vi "MASS_FLOW_METER.vi"(0 "ESD":bool, 3 "Wire cut":bool) -> (1 "MFM Flow Rate (Discharge)":dbl, 2 "MFM Flow Rate (Inlet)":dbl, 4 "MFM Total Kg (Discharge)":dbl format="%#_9g", 5 "MFM Total Kg (Inlet)":dbl format="%#_9g")   [LabVIEW 2014]
panel:
  out "Inlet MFM Total Kg Trend (Kg)":dbl(graph)
  out "Discharge MFM Total Kg Trend (Kg)":dbl(graph)
  out "Inlet MFM Flow Rate Trend (Kg/m2)":dbl(graph)
  out "Discharge MFM Flow Rate Trend (Kg/m2)":dbl(graph)
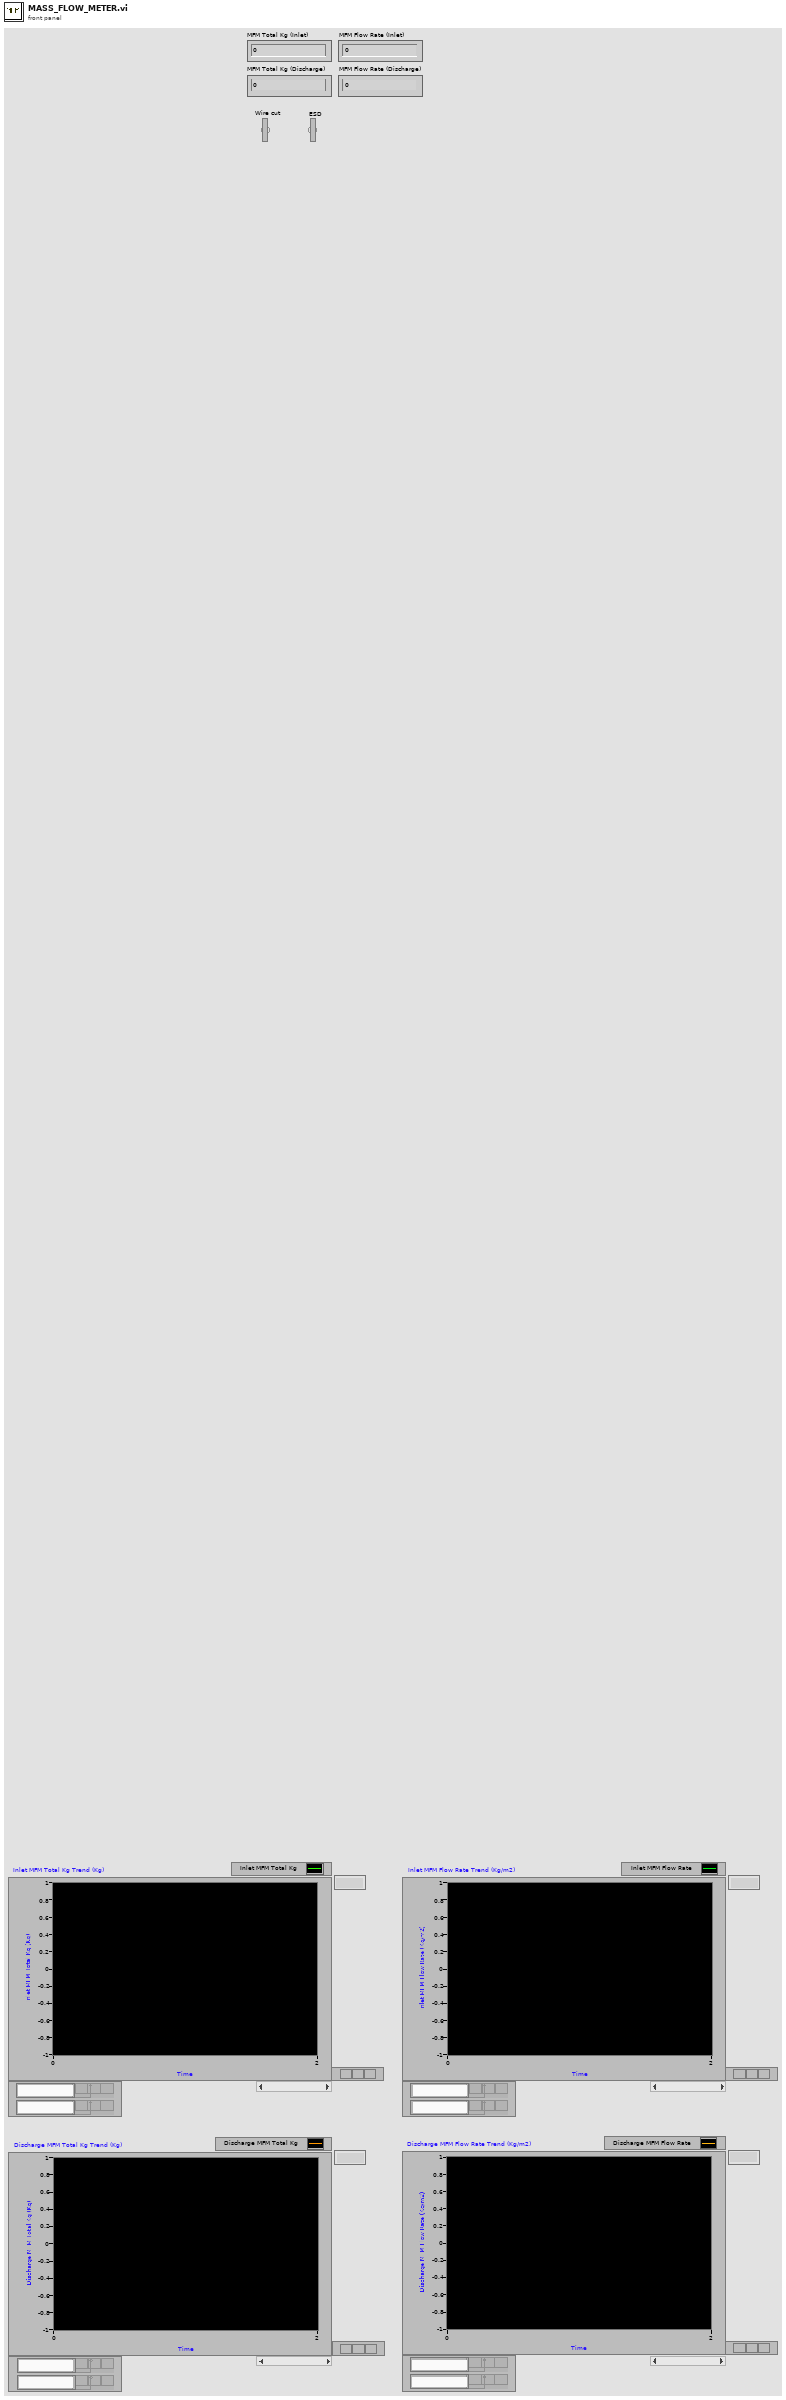
[diagram p1: front panel]
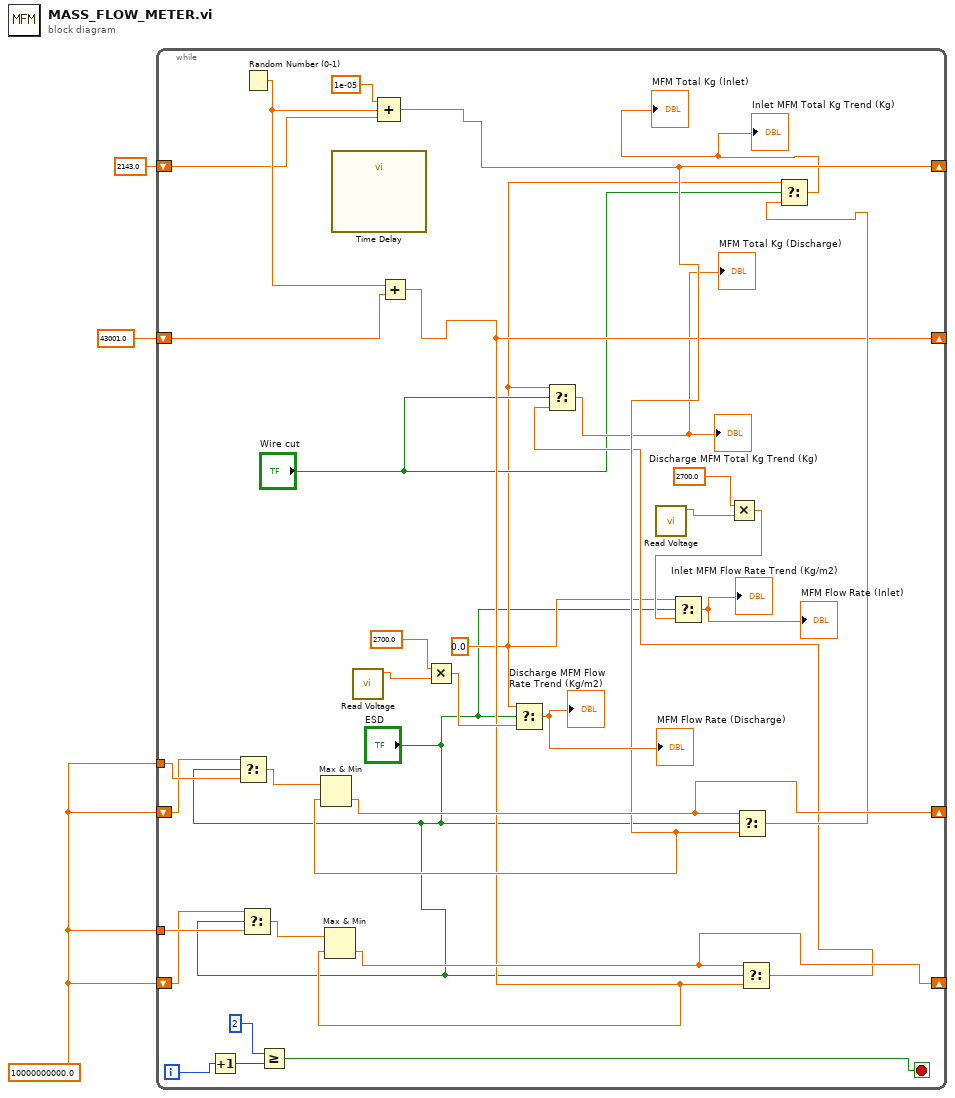
[diagram p0: block diagram]
diagram:
  w1 = 10000000000.0
  n1 = while {
    shift-right: [w16] -> _
    shift-left: 2143.0 -> [w29]
    shift-right: [w13] -> _
    shift-left: 43001.0 -> [w30]
    shift-right: [w28] -> _
    shift-left: w1 -> [w22]
    tunnel: w1 -> [w26]
    shift-right: [w23] -> _
    shift-left: w1 -> [w21]
    tunnel: w1 -> [w24]
    i -> [w8]
    stop <- w5 stop-if-true
    w9 = 0.0
    n2 = Increment(x=w8) -> (x+1=w7:i32)
    n3 = Select(t=w22, s="ESD", f=w26) -> (s? t:f=w27:dbl)
    n4 = Select(t=w21, s="ESD", f=w24) -> (s? t:f=w25:dbl)
    n5 = Random Number (0-1)() -> (number: 0 to 1=w36:dbl)
    n6 = Greater Or Equal?(x=2, y=w7) -> (x >= y?=w5:bool)
    n7 = call "Time Delay"() -> ()  [unwired: 11 in, 1 out]
    n8 = call "Read Voltage.vi"() -> ("voltage"=w31:dbl)  [unwired: 6 in, 1 out]
    n9 = Compound Arithmetic op=ADD(1e-05, w36, w29) -> (w16:dbl)
    n10 = Max & Min(x=w27, y=w16) -> (min(x,y)=w28:dbl)  [unwired: 1 out]
    n11 = Add(x=w36, y=w30) -> (x+y=w13:dbl)
    n12 = Max & Min(x=w25, y=w13) -> (min(x,y)=w23:dbl)  [unwired: 1 out]
    n13 = Multiply(x=2700.0, y=w31) -> (x*y=w20:dbl)
    n14 = Select(t=w9, s="ESD", f=w20) -> (s? t:f=→"Discharge MFM Flow Rate Trend (Kg/m2)" →"MFM Flow Rate (Discharge)":dbl)
    n15 = call "Read Voltage.vi"() -> ("voltage"=w33:dbl)  [unwired: 6 in, 1 out]
    n16 = Multiply(x=2700.0, y=w33) -> (x*y=w19:dbl)
    n17 = Select(t=w9, s="ESD", f=w19) -> (s? t:f=→"Inlet MFM Flow Rate Trend (Kg/m2)" →"MFM Flow Rate (Inlet)":dbl)
    n18 = Select(t=w28, s="ESD", f=w16) -> (s? t:f=w14:dbl)
    n19 = Select(t=w23, s="ESD", f=w13) -> (s? t:f=w12:dbl)
    n20 = Select(t=w9, s="Wire cut", f=w12) -> (s? t:f=→"Discharge MFM Total Kg Trend (Kg)" →"MFM Total Kg (Discharge)":dbl)
    n21 = Select(t=w9, s="Wire cut", f=w14) -> (s? t:f=→"MFM Total Kg (Inlet)" →"Inlet MFM Total Kg Trend (Kg)":dbl)
  }
